vi "Find Hardware Helper.vi"(7 "Framework":refnum<k21>, 8 "error in":errorcluster, 11 "Enumerator in":u64) -> (0 "error out":errorcluster, 2 "Found Resource":bool, 3 "Resource out":refnum<k20>)   [LabVIEW 2020, in "nisyscfg.lvlib"]
uses:
  <vilib>/nisyscfg/nisyscfg.lvlib
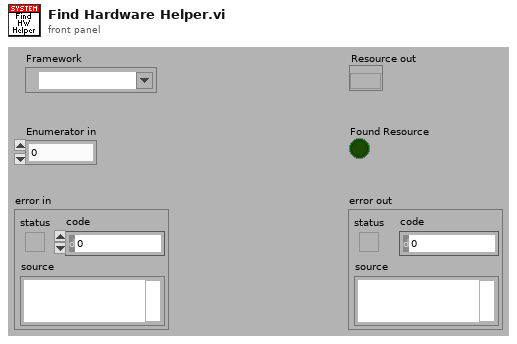
[diagram p1: front panel]
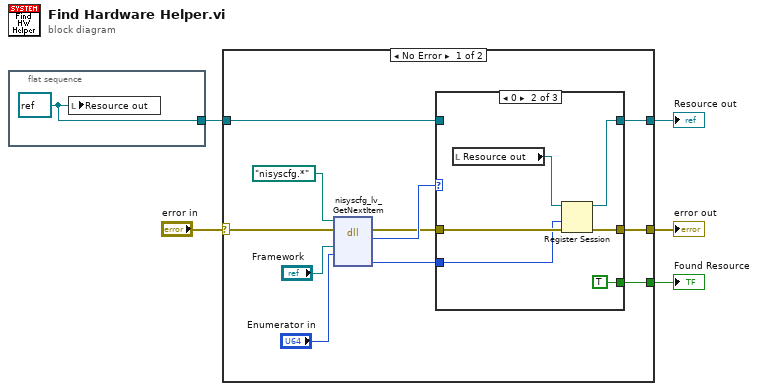
[diagram p0: block diagram]
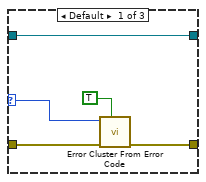
[diagram p2: hidden frame]
diagram:
  n1 = flat-sequence {
    tunnel: [w6] -> w2
    frame #0 {
      w6 = refnum<k20> refnum ("filter in")
      n2 = local write "Resource out"(w6) -> ()
    }
  }
  n3 = case shown="No Error" "error in" {
    selector: "error in" -> [w8 w32]
    tunnel: [w7 w32] -> w5
    tunnel: [w11 _] -> w4
    tunnel: [w10 w31] -> w3
    tunnel: w2 -> [w9 w31]
    frame No Error {
      n4 = dll-call lib="nisyscfg.*" fn="nisyscfg_lv_GetNextItem" label="GetNextItem"(path in=path "nisyscfg.*", error in=w8, "framework"="Framework", "itemsEnum"="Enumerator in") -> (error out=w13:errorcluster, "status"=w15:i32, "item"=w14:u64)  [unwired: 1 in, 4 out]
      n5 = case shown="0" w15 {
        selector: w15 -> [w18 _ _]
        tunnel: [_ TRUE _] -> w11
        tunnel: w14 -> [_ w26 _]
        tunnel: w13 -> [w20 w28 w30]
        tunnel: [w19 w27 w30] -> w7
        tunnel: [w22 w24 w29] -> w10
        tunnel: w9 -> [w22 _ w29]
        frame Default {
          n6 = call <vilib>:"Error Cluster From Error Code.vi"("show call chain? (False)"=TRUE, "error in (no error)"=w20, "error code (0)"=w18) -> ("error out"=w19:errorcluster)  [unwired: 6 out]
        }
        frame 0 {
          n7 = local read "Resource out"() -> (w25:refnum<k20>)
          n8 = Register Session(8:w28, 9:w26, 11:w25) -> (0:w27:errorcluster, 3:w24:refnum<k20>)  [unwired: 2 in]
        }
        frame 1 {
          # "This is S_FALSE which is\nthe enumerator end,\nbut it is not an error."
        }
      }
    }
    frame Error {
    }
  }
  "error out" <- w5
  "Resource out" <- w3
  "Found Resource" <- w4
